vi "Increment Plugin Iteration.vi"(8 "error in (no error)":errorcluster, 11 "Plugin in":refnum<class "Plugin.lvclass">) -> (0 "error out":errorcluster, 3 "Plugin out":refnum<class "Plugin.lvclass">)   [LabVIEW 2017, in "Data Sharing Framework Core.lvlib" / "Data Sharing Framework Engine.lvlib" / "Plugin.lvclass"]
uses:
  Plugin.lvclass
  Plugin.lvclass/Plugin.ctl
  Internal/Timing/Engine Timing.lvclass/Engine Timing.ctl
  Internal/Timing/Engine Timing.lvclass
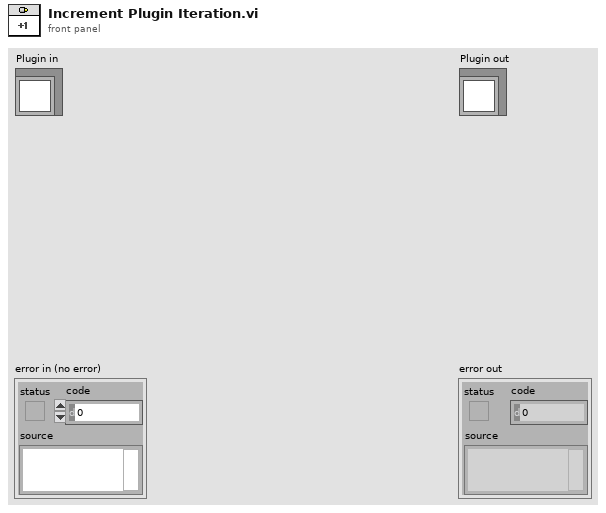
[diagram p1: front panel]
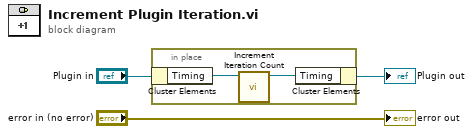
[diagram p0: block diagram]
diagram:
  n1 = in-place {
    n2 = in-place-cluster #1("Plugin in") -> ("Timing"=w5:refnum<class "Engine Timing.lvclass">)
    n3 = call "Increment Iteration Count.vi"("Timing in"=w5) -> ("Timing out"=w4:refnum<class "Engine Timing.lvclass">)  [unwired: 10 in]
    n4 = in-place-cluster #1("Timing"=w4) -> (→"Plugin out":refnum<class "Plugin.lvclass">)
  }
  "error out" <- "error in (no error)"
